vi "Add Image Data.vi"(7 "Control Info Cluster in":T1, 8 "error in (no error)":errorcluster, 10 "Ignore Image Data":bool, 11 "Control in":refnum<vi>) -> (0 "error out":errorcluster, 3 "Control out":refnum<vi>, 5 "Control Info Cluster out":T1)   [LabVIEW 2023, in "VIDoc Parsing.lvlib"]
doc: "Optionally adds the Control Image Data to the Control Info Cluster."
uses:
  VIDoc Parsing.lvlib
  TypeDefs/Controls Info Cluster.ctl
  <vilib>/picture/picture.llb/imagedata.ctl
  <vilib>/Utility/miscctls.llb/LVKeyTypeDef.ctl
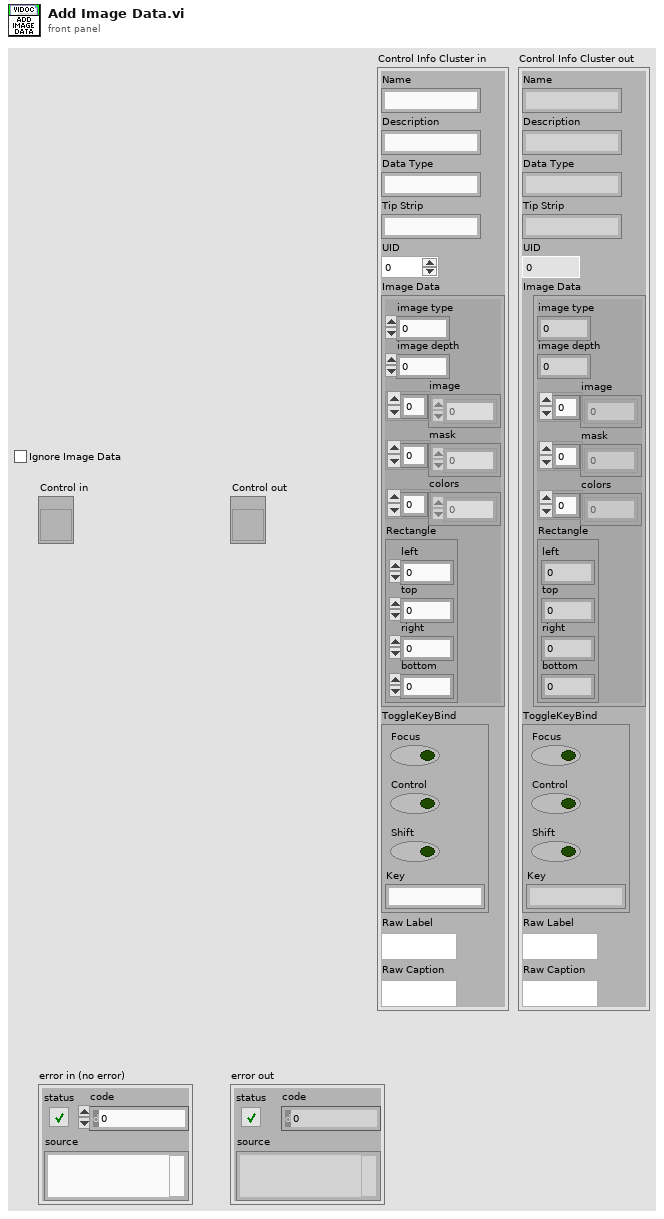
[diagram p1: front panel]
types:
  T1 = typedef "VIDoc Parsing.lvlib/Controls Info Cluster.ctl" = cluster{"Name":string, "Description":string, "Data Type":string, "Tip Strip":string, "UID":i32, "Image Data":T2, "ToggleKeyBind":T3, "Raw Label":string, "Raw Caption":string}
  T2 = typedef "imagedata.ctl" = cluster{"image type":i32, "image depth":i32, "image":u8[], "mask":u8[], "colors":u32[], "Rectangle":cluster{"left":i16, "top":i16, "right":i16, "bottom":i16}}
  T3 = typedef "LVKeyTypeDef.ctl" = cluster{"Focus":bool, "Control":bool, "Shift":bool, "Key":string}
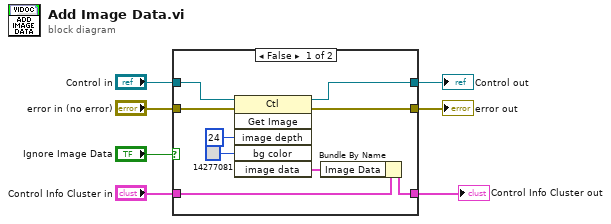
[diagram p0: block diagram]
diagram:
  n1 = case shown="False" "Ignore Image Data" {
    tunnel: [w15 w18] -> w7
    tunnel: "Control in" -> [w14 w18]
    tunnel: "error in (no error)" -> [w13 w19]
    tunnel: [w12 w19] -> w4
    tunnel: "Control Info Cluster in" -> [w10 w17]
    tunnel: [w8 w17] -> w1
    frame False {
      n2 = invoke class="Ctl" method="Get Image"(reference=w14, error in=w13, "image depth"=24 ("Image Depth"), "bg color"=u32 14277081 ("Color Box")) -> (reference out=w15:refnum<vi>, error out=w12:errorcluster, "image data"=w9:T2)  [unwired: 2 in, 3 out]
      n3 = Bundle By Name(cluster=w10, "Image Data"=w9) -> (w8:T1)
    }
    frame True {
    }
  }
  "Control out" <- w7
  "error out" <- w4
  "Control Info Cluster out" <- w1
